vi "SLL DE Wait for DO Response.vi"(8 "Error In":errorcluster, 9 "Timeout (Sec)":dbl=5.0, 10 "Executed For?":string, 11 "Check Response?":bool) -> (0 "error out":errorcluster, 3 "Done?":bool)   [LabVIEW 2013]
uses:
  Controls/SLL DE DO Response LV2Global Options.ctl
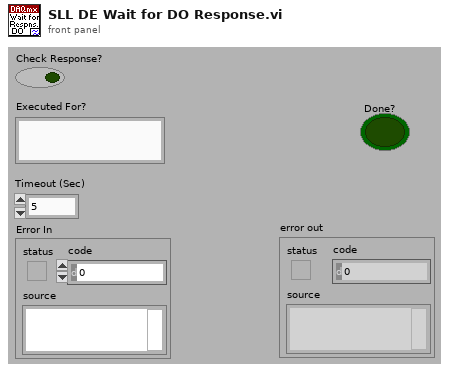
[diagram p1: front panel]
types:
  T1 = typedef "SLL DE DO Response LV2Global Options.ctl" = enum16{"Initialize", "Send Response", "Check Response", "Close"}
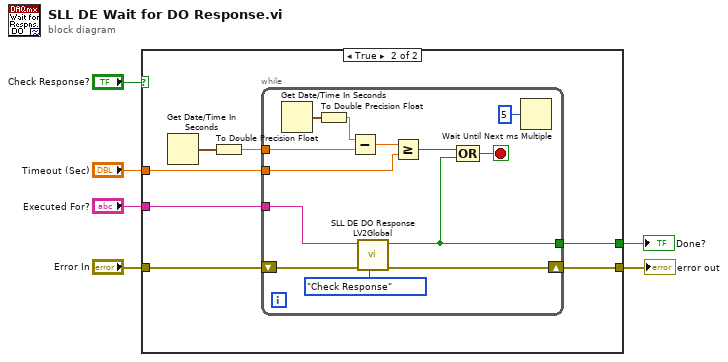
[diagram p0: block diagram]
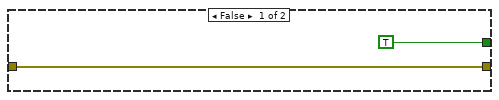
[diagram p2: hidden frame]
diagram:
  n1 = case shown="True" "Check Response?" {
    tunnel: "Executed For?" -> [_ w14]
    tunnel: "Error In" -> [w7 w13]
    tunnel: [w7 w12] -> _
    tunnel: [TRUE ("Found?") w11] -> w2
    tunnel: "Timeout (Sec)" -> [_ w8]
    frame False {
    }
    frame True {
      n2 = Get Date/Time In Seconds() -> (seconds since 1Jan1904=w10:timestamp)
      n3 = To Double Precision Float(number=w10) -> (double precision float=w9:dbl)
      n4 = while {
        tunnel: w14 -> [w27]
        shift-right: [w25] -> w12
        shift-left: w13 -> [w26]
        tunnel: [w17] -> w11
        tunnel: w9 -> [w21]
        tunnel: w8 -> [w15]
        stop <- w16 stop-if-true
        n5 = Get Date/Time In Seconds() -> (seconds since 1Jan1904=w22:timestamp)
        n6 = To Double Precision Float(number=w22) -> (double precision float=w19:dbl)
        n7 = Subtract(x=w19, y=w21) -> (x-y=w20:dbl)
        n8 = call "SLL DE DO Response LV2Global.vi"("Option"=SLL_DE_DO_Response_LV2Global_Options."Check Response", "Error in (no error)"=w26, "Executed For?"=w27) -> ("Error out"=w25:errorcluster, "Found?"=w17:bool)  [unwired: 7 in]
        n9 = Greater Or Equal?(x=w20, y=w15) -> (x >= y?=w18:bool)
        n10 = Compound Arithmetic op=OR(w18, w17) -> (w16:bool)
        n11 = Wait Until Next ms Multiple(millisecond multiple=u32 5) -> ()  [unwired: 1 out]
      }
    }
  }
  "Done?" <- w2
  "error out" <- "Error In"
